vi "Read Temp Humidity.vi"(8 "error in (no error)":errorcluster, 11 "Grove Temperature Humidity Sensor DH20 in":refnum<class "Grove Temperature Humidity Sensor DH20.lvclass">) -> (0 "error out":errorcluster, 1 "Humidity":dbl, 2 "Temperature":dbl, 3 "Grove Temperature Humidity Sensor DH20 out":refnum<class "Grove Temperature Humidity Sensor DH20.lvclass">)   [LabVIEW 2020, in "CTI-Peripheral.lvlib" / "Grove Temperature Humidity Sensor DH20.lvclass"]
uses:
  Grove Temperature Humidity Sensor DH20.lvclass
  Grove Temperature Humidity Sensor DH20.lvclass/Grove Temperature Humidity Sensor DH20.ctl
  CTI/I2C Connection/I2C Connection.lvclass/I2C Connection.ctl
  CTI/Session/I2C Write Data.vi
  CTI/Session/I2C Read Data.vi
  CTI/I2C Connection/I2C Connection.lvclass
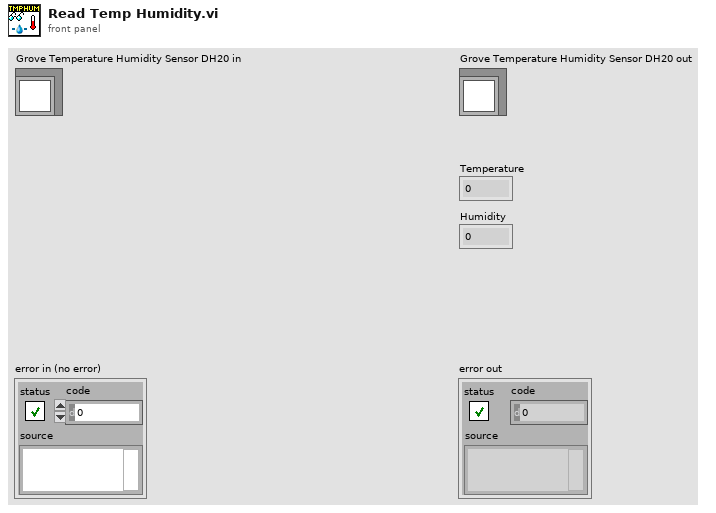
[diagram p1: front panel]
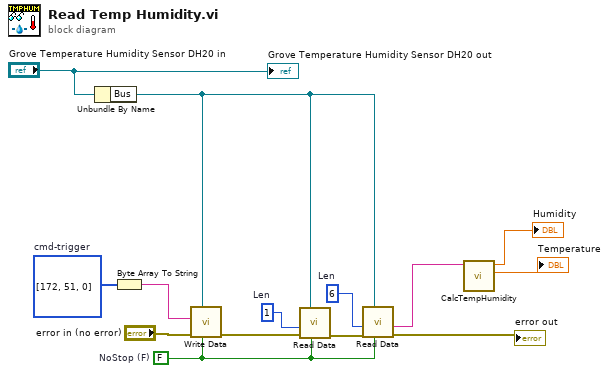
[diagram p0: block diagram]
diagram:
  w3 = u8 6  # Len
  w10 = u8[] [172, 51, 0]  # cmd-trigger
  w8 = FALSE  # NoStop (F)
  w12 = u8 1  # Len
  n1 = Unbundle By Name("Grove Temperature Humidity Sensor DH20 in") -> ("Bus"=w6:refnum<class "I2C Connection.lvclass">)
  n2 = Byte Array To String(unsigned byte array=w10) -> (string=w9:string)
  n3 = call "Write Data.vi"("NoStop (F)"=w8, "I2C Connection"=w6, "error in (no error)"="error in (no error)", "Data"=w9) -> ("error out"=w11:errorcluster)  [unwired: 7 in]
  n4 = call "Read Data.vi"("NoStop (F)"=w8, "I2C Connection"=w6, "error in (no error)"=w11, "Len"=w12) -> ("error out"=w7:errorcluster)  [unwired: 6 in, 1 out]
  n5 = call "Read Data.vi"("NoStop (F)"=w8, "I2C Connection"=w6, "error in (no error)"=w7, "Len"=w3) -> ("error out"=→"error out":errorcluster, "Data"=w4:string)  [unwired: 6 in]
  n6 = call "CalcTempHumidity.vi"("Data"=w4) -> ("Temperature (°C)"=→"Temperature":dbl, "RHumidity%"=→"Humidity":dbl)  [unwired: 9 in]
  "Grove Temperature Humidity Sensor DH20 out" <- "Grove Temperature Humidity Sensor DH20 in"
